vi "自动配置的串口通信组件(Slave).vi"(5 "error in":errorcluster) -> (11 "Stop":bool, 19 "error out":errorcluster)   [LabVIEW 2013]
uses:
  <vilib>/Instr/_visa.llb/VISA Configure Serial Port (Instr).vi
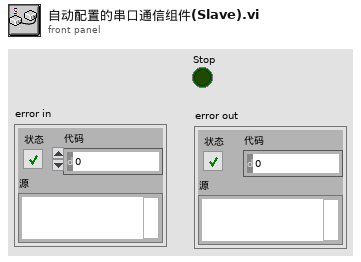
[diagram p1: front panel]
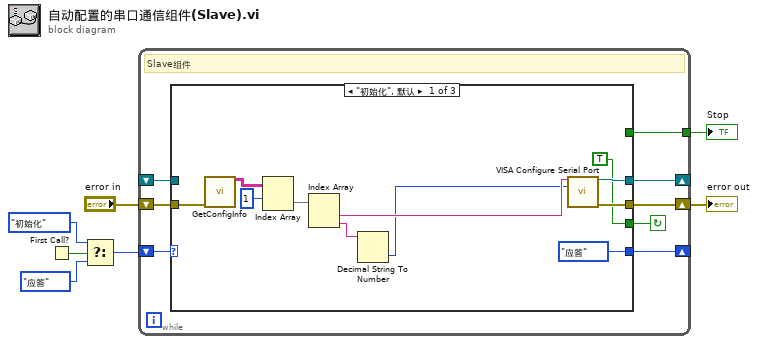
[diagram p0: block diagram]
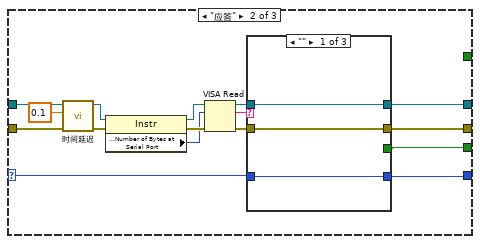
[diagram p2: hidden frame]
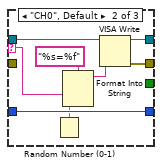
[diagram p3: hidden frame]
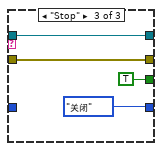
[diagram p4: hidden frame]
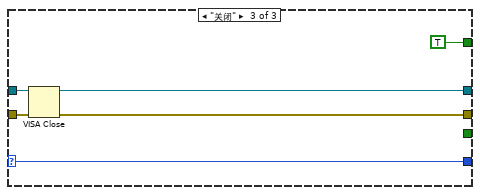
[diagram p5: hidden frame]
diagram:
  n1 = First Call?() -> (First Call?: T/F=w7:bool)
  n2 = Select(t=enum16{"初始化", "应答", "关闭"}."初始化" ("枚举"), s=w7, f=enum16{"初始化", "应答", "关闭"}."应答" ("枚举")) -> (s? t:f=w6:enum16{"初始化", "应答", "关闭"})
  n3 = while {
    shift-right: [w15] -> w3
    shift-left: "error in" -> [w13]
    shift-right: [w14] -> _
    shift-left: _ -> [w12]
    shift-right: [w11] -> _
    shift-left: w6 -> [w10]
    tunnel: [w8] -> w1
    stop <- w9 continue-if-true
    # "Slave组件"
    n4 = case shown="\"初始化\", 默认" w10 {
      selector: w10 -> [_ w34 w58]
      tunnel: [w26 w30 w59] -> w14
      tunnel: [w25 w28 w60] -> w15
      tunnel: w13 -> [w22 w36 w61]
      tunnel: w12 -> [_ w35 w59]
      tunnel: [TRUE w29 _] -> w9
      tunnel: [enum16{"初始化", "应答", "关闭"}."应答" ("枚举") w33 w58] -> w11
      tunnel: [_ _ TRUE] -> w8
      frame "初始化", Default {
        n5 = call "GetConfigInfo.vi"("error in (no error)"=w22) -> ("串口配置"=w19:string[][])  [unwired: 17 in, 1 out]
        n6 = Index Array(array=w19, index (row)=1 ("索引 (行)")) -> (element=w20:string[])  [unwired: 1 in]
        n7 = Index Array(array=w20) -> (element #1=w17:string, element #2=w21:string)  [unwired: 2 in]
        n8 = Decimal String To Number(string=w21) -> (number=w16:i32)  [unwired: 2 in, 1 out]
        n9 = call-poly "VISA Configure Serial Port"("VISA resource name"=w17, "baud rate (9600)"=w16) -> ("VISA resource name out"=w26:refnum<visa-resource-name>, "error out"=w25:errorcluster)  [unwired: 12 in]
      }
      frame "应答" {
        n10 = call "时间延迟"("error in (no error)"=w36, "Delay Time (s)"=0.1) -> ("error out"=w38:errorcluster)  [unwired: 9 in]
        n11 = property class="Instr"(reference=w35, error in=w38) -> (reference out=w39:refnum<visa-resource-name>, error out=w41:errorcluster, "Serial Settings:Number of Bytes at Serial Port"=w40:u32)
        n12 = VISA Read(VISA resource name=w39, byte count=w40, error in (no error)=w41) -> (VISA resource name out=w31:refnum<visa-resource-name>, read buffer=w32:string, error out=w27:errorcluster)  [unwired: 1 out]
        n13 = case shown="\"\"" w32 {
          selector: w32 -> [_ w46 _]
          tunnel: w31 -> [w43 w52 w56]
          tunnel: [w43 w51 w56] -> w30
          tunnel: [w42 w50 w53] -> w28
          tunnel: [_ _ TRUE] -> w29
          tunnel: [w44 w49 enum16{"初始化", "应答", "关闭"}."关闭" ("枚举")] -> w33
          tunnel: w34 -> [w44 w49 _]
          tunnel: w27 -> [w42 _ w53]
          frame "" {
          }
          frame "CH0", Default {
            n14 = Random Number (0-1)() -> (number: 0 to 1=w47:dbl)
            n15 = Format Into String(format string="%s=%f" ("格式字符串"), w46, w47) -> (resulting string=w45:string)  [unwired: 2 in, 1 out]
            n16 = VISA Write(VISA resource name=w52, write buffer=w45) -> (VISA resource name out=w51:refnum<visa-resource-name>, error out=w50:errorcluster)  [unwired: 1 in, 1 out]
          }
          frame "Stop" {
          }
        }
      }
      frame "关闭" {
        n17 = VISA Close(VISA resource name=w59, error in (no error)=w61) -> (error out=w60:errorcluster)
      }
    }
  }
  "error out" <- w3
  "Stop" <- w1
